vi "Camera Global Data.vi"() -> ()   [LabVIEW 2013]
panel:
  in  "Camera Sonar":dbl
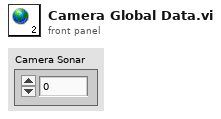
[diagram p1: front panel]
diagram:
